vi "Run_try2.vi"(7 "Team Index":i32, 8 "Column":i32, 9 "Row":i32, 10 "View":i32[](array[numeric]) caption="View (Team Index, -1: empty)", 11 "Atom In":refnum<class "Atom.lvclass">) -> (0 "Replicated":refnum<class "Square.lvclass">, 1 "Direction":T1, 2 "Action":T2=enum."Replicate", 3 "Square Out":refnum<class "Square.lvclass">)   [LabVIEW 2020, in "Atom.lvclass"]
uses:
  Atom.lvclass
  C:/dev/IlluminatedG/sol-squarebattle/Square/Square.lvclass
  Square/Square.lvclass
  Type Defs/Action Enum.ctl
  Type Defs/Direction Enum.ctl
  Atom.lvclass/Atom.ctl
  Type Defs/SB Type Defs.lvlib
panel:
  # "NW\nN\nNE\nE\nSE\nS\nSW\nW"
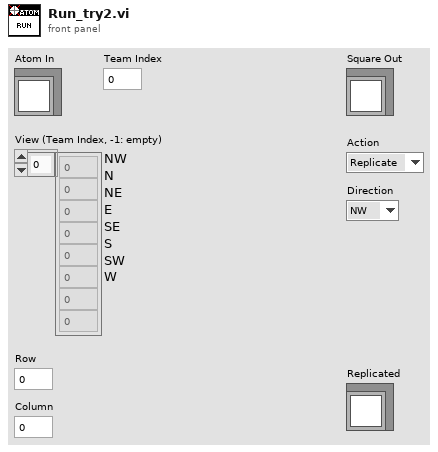
[diagram p1: front panel]
types:
  T1 = typedef "SB Type Defs.lvlib/Direction Enum.ctl" = enum16{"NW", "N", "NE", "E", "SE", "S", "SW", "W"}
  T2 = typedef "SB Type Defs.lvlib/Action Enum.ctl" = enum16{"Wait", "Move", "Attack", "Replicate"}
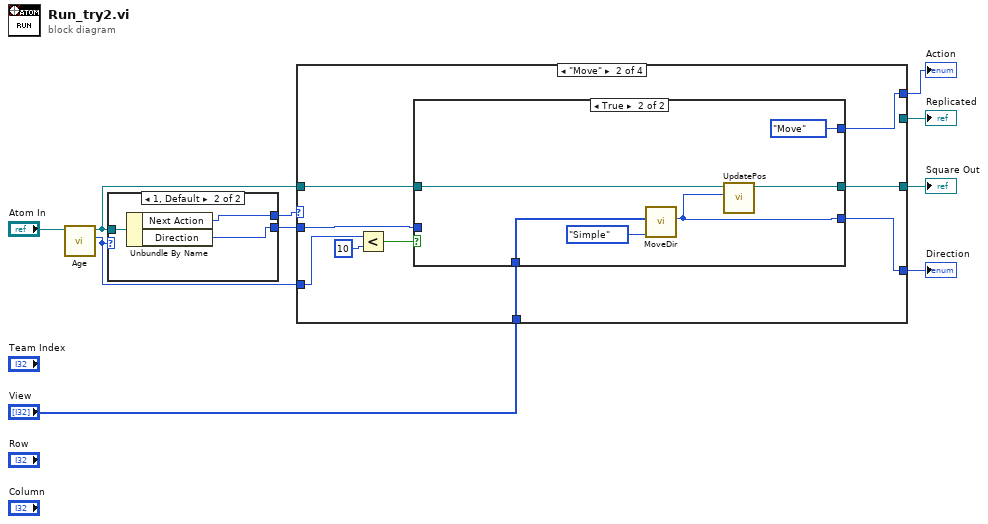
[diagram p0: block diagram]
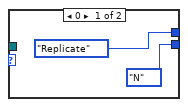
[diagram p2: hidden frame]
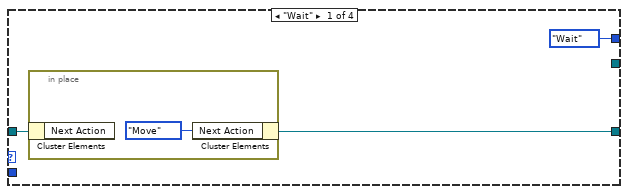
[diagram p3: hidden frame]
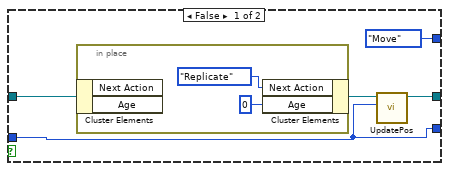
[diagram p4: hidden frame]
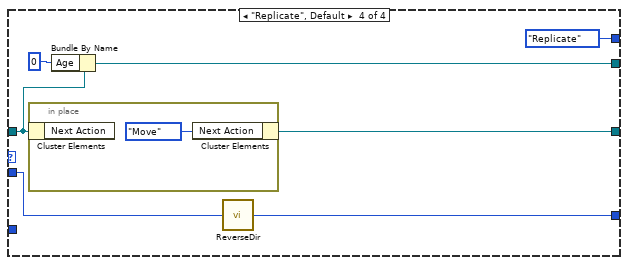
[diagram p6: hidden frame]
diagram:
  n1 = call "Age.vi"("Atom In"="Atom In") -> ("Current Age"=w2:i32, "Atom Out"=w3:refnum<class "Atom.lvclass">)  [unwired: 9 in]
  n2 = case shown="1, Default" w2 {
    tunnel: [Action_Enum."Replicate" ("Action") w15] -> w9
    tunnel: [Direction_Enum."N" ("Direction") w14] -> w6
    tunnel: w3 -> [_ w13]
    frame 0 {
    }
    frame 1, Default {
      n3 = Unbundle By Name(w13) -> ("Next Action"=w15:T2, "Direction"=w14:T1)
    }
  }
  n4 = case shown="\"Move\"" w9 {
    tunnel: [w16 w24 w42 w44] -> w10
    tunnel: w3 -> [w17 w25 w42 w45]
    tunnel: [Action_Enum."Wait" ("Action") w28 _ Action_Enum."Replicate" ("Action")] -> w8
    tunnel: [_ w20 _ w48] -> w7
    tunnel: w6 -> [_ w23 _ w47]
    tunnel: [_ _ _ w43] -> w5
    tunnel: w2 -> [_ w22 _ _]
    tunnel: "View" -> [_ w21 _ _]
    frame "Wait" {
      n5 = in-place {
        n6 = in-place-cluster #1(w17) -> ()  [unwired: 1 out]
        n7 = in-place-cluster #1("Next Action"=Action_Enum."Move") -> (w16:refnum<class "Atom.lvclass">)
      }
    }
    frame "Move" {
      n8 = Less?(x=w22, y=10) -> (x < y?=w26:bool)
      n9 = case shown="True" w26 {
        tunnel: [Action_Enum."Move" ("Action") Action_Enum."Move" ("Action")] -> w28
        tunnel: w25 -> [w32 w41]
        tunnel: [w30 w39] -> w24
        tunnel: w23 -> [w29 _]
        tunnel: w21 -> [_ w38]
        tunnel: [w29 w36] -> w20
        frame False {
          n10 = in-place {
            n11 = in-place-cluster #2(w32) -> ()  [unwired: 2 out]
            n12 = in-place-cluster #2("Next Action"=Action_Enum."Replicate", "Age"=0) -> (w31:refnum<class "Atom.lvclass">)
          }
          n13 = call "UpdatePos.vi"("Direction"=w29, "Atom In"=w31) -> ("Atom Out"=w30:refnum<class "Atom.lvclass">)  [unwired: 9 in]
        }
        frame True {
          n14 = call "MoveDir.vi"("Type"=enum16{"Random", "Simple"}."Simple", "View"=w38) -> ("Direction"=w36:T1)  [unwired: 7 in, 2 out]
          n15 = call "UpdatePos.vi"("Direction"=w36, "Atom In"=w41) -> ("Atom Out"=w39:refnum<class "Atom.lvclass">)  [unwired: 9 in]
        }
      }
    }
    frame "Attack" {
    }
    frame "Replicate", Default {
      n16 = in-place {
        n17 = in-place-cluster #3(w45) -> ()  [unwired: 1 out]
        n18 = in-place-cluster #3("Next Action"=Action_Enum."Move" ("Action")) -> (w44:refnum<class "Atom.lvclass">)
      }
      n19 = Bundle By Name(cluster=w45, "Age"=0) -> (w43:refnum<class "Atom.lvclass">)
      n20 = call "ReverseDir.vi"("Direction"=w47) -> ("Direction Out"=w48:T1)
    }
  }
  "Square Out" <- w10
  "Action" <- w8
  "Direction" <- w7
  "Replicated" <- w5
